vi "Using_the_gps.vi"() -> ()   [LabVIEW 2009]
uses:
  Novatel GPS new.llb/GPSINS output.ctl
panel:
  out "GPS Status":T1
  out "GPS cluster":T2 {"Northing" format="%#.2f"; "Easting" format="%#.2f"}
  in  "stop":bool
  out "GPS Data":T3 {"Easting" format="%#.10f"; "Northing" format="%#.10f"}
  in  "GPS Com":refnum<visa-resource-name>
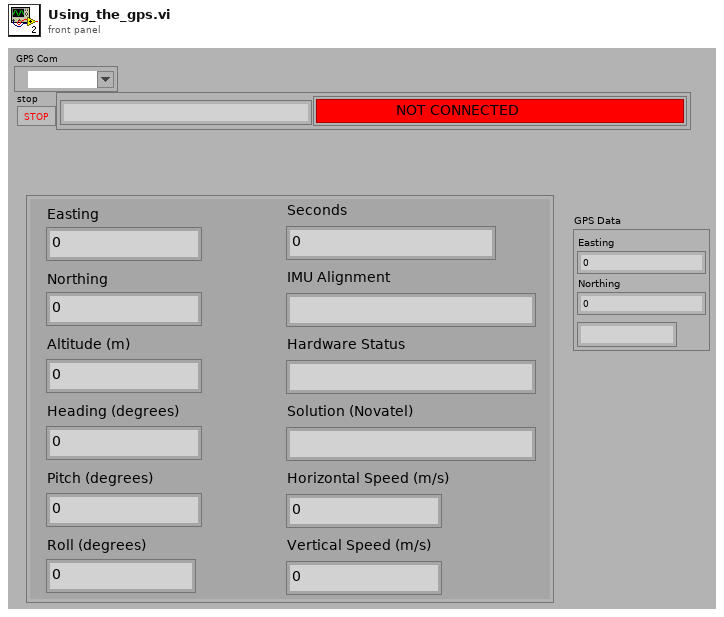
[diagram p1: front panel]
types:
  T1 = cluster{"GPS Connected":bool, "GPS Connect Status":string}
  T2 = typedef "GPSINS output.ctl" = cluster{"Easting ":dbl, "Northing":dbl, "Horizontal Speed (m/s)":dbl, "Heading (degrees)":dbl, "Pitch (degrees)":dbl, "Roll (degrees)":dbl, "IMU Alignment":string, "Hardware Status":string, "Solution (Novatel)":string, "Altitude (m)":dbl, "Vertical Speed (m/s)":dbl, "Seconds":u32}
  T3 = cluster{"Easting":dbl, "Northing":dbl, "Status":string}
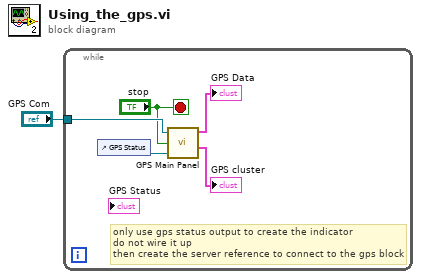
[diagram p0: block diagram]
diagram:
  n1 = while {
    tunnel: "GPS Com" -> [w6]
    stop <- "stop" stop-if-true
    # "only use gps status output to create the indicator\ndo not wire it up\nthen create the server reference to connect to the gps block"
    n2 = control-ref of="GPS Status"() -> (w2:refnum<vi>)
    n3 = call "GPS Main Panel.vi"("GPS Status Ref"=w2, "stop"="stop", "GPS Com"=w6) -> ("GPS cluster"=→"GPS cluster":T2, "GPS Data"=→"GPS Data":T3)  [unwired: 3 in, 1 out]
  }
